vi "GlobalDataAddress.vi"(4 "Data IDs In":dbl[](array[numeric]), 5 "Data Names In":string[](array[string]), 6 "Element index":u16, 7 "Function select":string) -> (0 "Data ID":u16, 1 "Data name":string, 2 "Data ID Out":dbl[](array[numeric]), 3 "Data Names Out":string[](array[string]))   [LabVIEW 2013]
uses:
  GlobalParamSize.vi
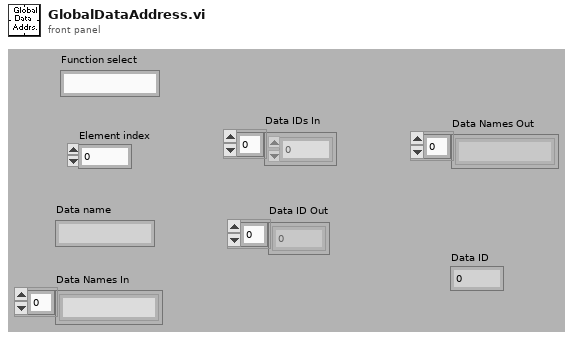
[diagram p1: front panel]
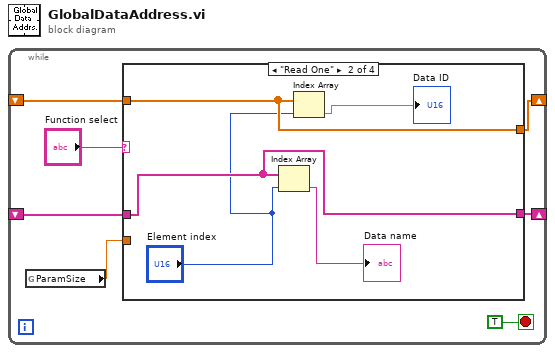
[diagram p0: block diagram]
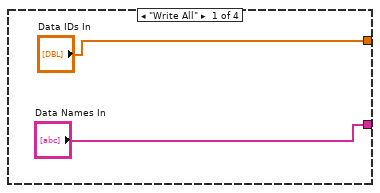
[diagram p2: hidden frame]
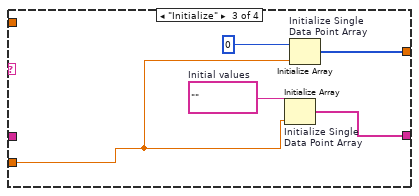
[diagram p3: hidden frame]
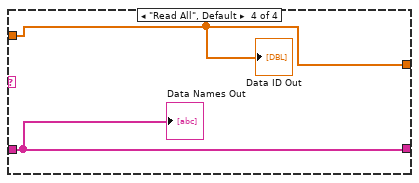
[diagram p4: hidden frame]
diagram:
  n1 = while {
    shift-right: [w5] -> _
    shift-left: _ -> [w4]
    shift-right: [w3] -> _
    shift-left: _ -> [w2]
    stop <- TRUE stop-if-true
    n2 = global read "GlobalParamSize.vi" "ParamSize"() -> (w1:dbl)
    n3 = case shown="\"Read One\"" "Function select" {
      tunnel: w1 -> [_ _ w17 _]
      tunnel: ["Data Names In" w13 w18 w21] -> w5
      tunnel: w4 -> [_ w13 _ w21]
      tunnel: ["Data IDs In" w12 w15 w20] -> w3
      tunnel: w2 -> [_ w12 _ w20]
      frame "Write All" {
      }
      frame "Read One" {
        n4 = Index Array(array=w13, index="Element index") -> (element=→"Data name":string)
        n5 = Index Array(array=w12, index="Element index") -> (element=→"Data ID":dbl)
      }
      frame "Initialize" {
        w19 = ""  # Initial values
        n6 = Initialize Array "Initialize Single\nData Point Array"(w19, w17) -> (w18:string[])
        n7 = Initialize Array "Initialize Single\nData Point Array"(0, w17) -> (w15:i32[])
      }
      frame "Read All", Default {
        "Data Names Out" <- w21
        "Data ID Out" <- w20
      }
    }
  }
